vi "Analysator Index by Name.vi"(7 "byName":bool, 11 "Analysator":string) -> (3 "Analysator Index":i32)   [LabVIEW 2020, in "System Einstellungen V2.lvlib"]
uses:
  System Einstellungen V2.lvlib
  Aktion FGV SystemEinstellungenV2.ctl
  AnalysatorDefinition.ctl
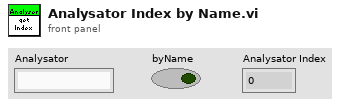
[diagram p1: front panel]
types:
  T1 = typedef "System Einstellungen V2.lvlib/AnalysatorDefinition.ctl" = cluster{"Analysator":string, "Name für Protokoll":string, "Type":string, "Seriennummer":string}
  T2 = typedef "System Einstellungen V2.lvlib/Aktion FGV SystemEinstellungenV2.ctl" = enum16{"lesen", "Analysatoren schreiben", "Analysator ändern", "Analysatoren löschen", "laden", "speichern", "Untertitel", "Analysatoren", "Neue Analysatoren", "Gasteiler schreiben", "Gasteiler ändern", "Gasteiler löschen", "Gasteiler", "Gasteiler exportieren", "Gasteiler importieren"}
  T3 = typedef "LVComboBoxStrsAndValuesArrayTypeDef.ctl" = cluster{"String":string, "Value":string}[]
  T4 = cluster{"AnalysatorDefinitionListe":T1[], "AnalysatorDefinitionTextListe":string[][], "Analysatoren Strings And Values[]":T3}
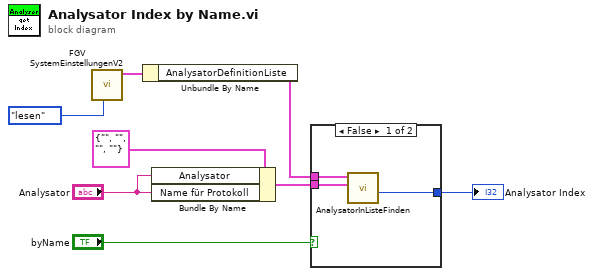
[diagram p0: block diagram]
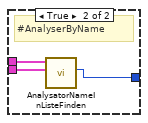
[diagram p2: hidden frame]
diagram:
  n1 = call "FGV SystemEinstellungenV2.vi"("Aktion"=Aktion_FGV_SystemEinstellungenV2."lesen") -> ("Analysatoren"=w7:T4)  [unwired: 5 in, 5 out]
  n2 = Unbundle By Name(w7) -> ("AnalysatorDefinitionListe"=w2:T1[])
  n3 = Bundle By Name(cluster=T1 {"Analysator"="", "Name für Protokoll"="", "Type"="", "Seriennummer"=""} ("AnalysatorDefinition"), "Analysator"="Analysator", "Name für Protokoll"="Analysator") -> (w3:T1)
  n4 = case shown="False" "byName" {
    tunnel: w2 -> [w11 w14]
    tunnel: w3 -> [w10 w13]
    tunnel: [w9 w12] -> w1
    frame False {
      n5 = call "AnalysatorInListeFinden.vi"("AnalysatorDefinition"=w10, "AnalysatorListe"=w11) -> ("Index"=w9:i32)  [unwired: 6 in, 3 out]
    }
    frame True {
      # "#AnalyserByName"
      n6 = call "AnalysatorNameInListeFinden.vi"("AnalysatorDefinition"=w13, "AnalysatorListe"=w14) -> ("Index"=w12:i32)  [unwired: 6 in, 3 out]
    }
  }
  "Analysator Index" <- w1
